vi "SettingsGUI.vi"() -> ()   [LabVIEW 2014]
panel:
  in  "Control":T1(tab)
  in  "Size (um)":dbl(slide) scale=0.0..10.0
  in  "Centroid":bool
  in  "Angular Mag.":dbl[unit]
  in  "Objective EFL":dbl[unit]
  in  "Tree":string(tree)
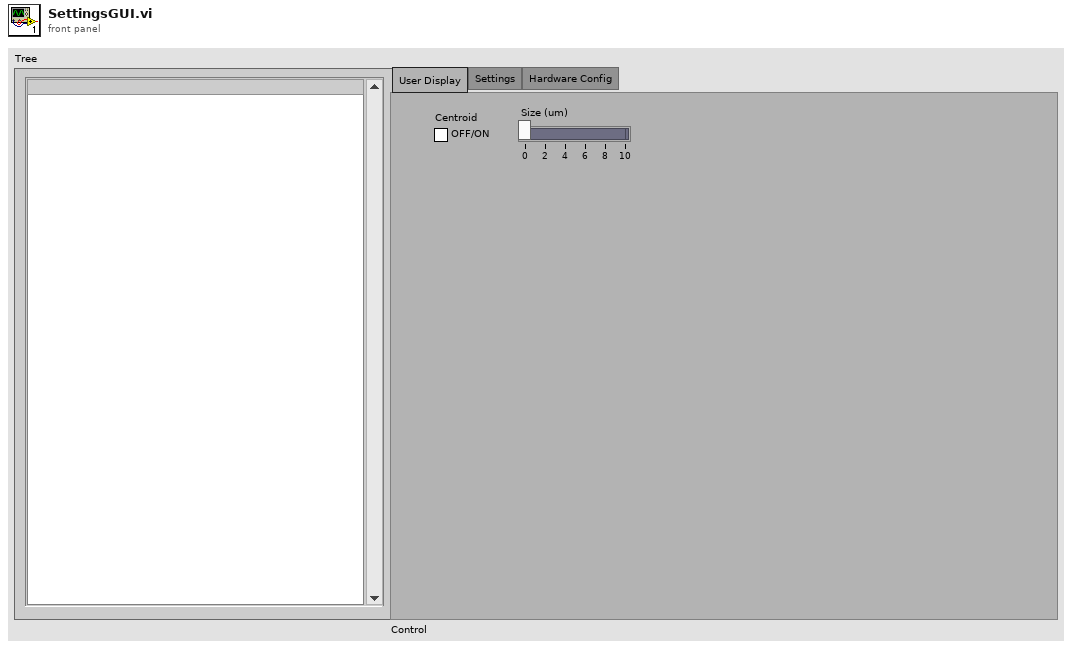
[diagram p1: front panel]
types:
  T1 = enum32{"User Display", "Settings", "Hardware Config"}
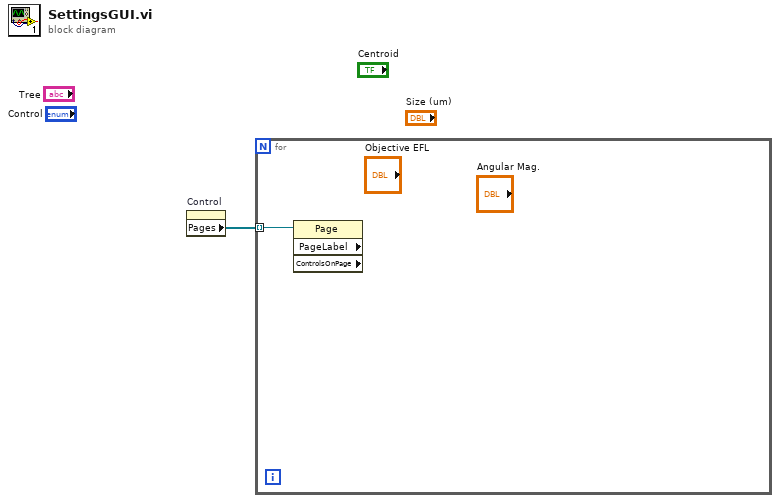
[diagram p0: block diagram]
diagram:
  n1 = property on="Control" class="TabCtl (strict)"() -> ("Pages"=w1:refnum<vi>[])  [unwired: 2 in, 2 out]
  n2 = for {
    tunnel: w1 -> [w2] mode=indexing
    n3 = property class="Page" props=["PageLabel", "ControlsOnPage"](reference=w2) -> ()  [unwired: 1 in, 4 out]
  }
